vi "DestroySelfReference.vi"(8 "error in (no error)":errorcluster, 11 "Measurement.PhotocurrentMapping":refnum<class "Measurement.PhotocurrentMapping.lvclass">) -> (0 "error out":errorcluster, 3 "Measurement.PhotocurrentMapping out":refnum<class "Measurement.PhotocurrentMapping.lvclass">)   [LabVIEW 2017, in "Measurement.PhotocurrentMapping.lvclass"]
doc: "JKI State Machine Objects (SMO) 1.0.0.5\nJKI - JKI\nCopyright (c) 2016, JKI"
uses:
  Measurement.PhotocurrentMapping.lvclass
  Measurement.PhotocurrentMapping.lvclass/Measurement.PhotocurrentMapping.ctl
  Measurement/Measurement.lvclass
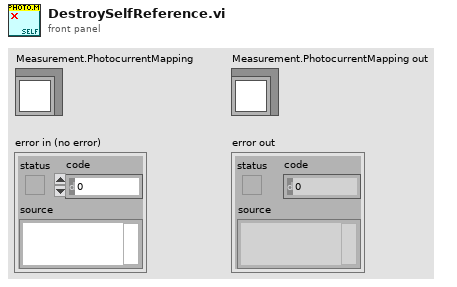
[diagram p1: front panel]
types:
  T1 = typedef "Measurement.PhotocurrentMapping.lvclass/PrivateData--Ref.ctl" = refnum<data-value>
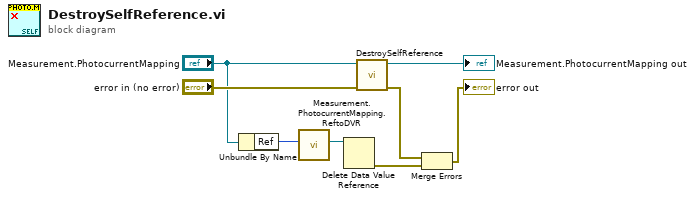
[diagram p0: block diagram]
diagram:
  n1 = Unbundle By Name("Measurement.PhotocurrentMapping") -> ("Ref"=w2:u32)
  n2 = call "Measurement.PhotocurrentMapping.ReftoDVR.vi"("Ref"=w2) -> ("Ref"=w1:T1)  [unwired: 10 in]
  n3 = Delete Data Value Reference(data value reference=w1) -> (error out=w5:errorcluster)  [unwired: 1 in, 1 out]
  n4 = call-parent "DestroySelfReference.vi"("error in (no error)"="error in (no error)", "Measurement"="Measurement.PhotocurrentMapping") -> ("error out"=w4:errorcluster, "Measurement out"=→"Measurement.PhotocurrentMapping out":refnum<class "Measurement.PhotocurrentMapping.lvclass">)  [unwired: 8 in]
  n5 = Merge Errors(w4, w5) -> (→"error out":errorcluster)
